vi "Register Worker.vi"(8 "error in (no error)":errorcluster, 10 "Worker":refnum<class "Job Handler.lvclass">, 11 "Mock Worker Processor In":refnum<class "Mock Job Dispatcher.lvclass">) -> (0 "error out":errorcluster, 3 "Mock Worker Processor Out":refnum<class "Mock Job Dispatcher.lvclass">)   [LabVIEW 2020, in "Mock Job Dispatcher.lvclass"]
uses:
  Mock Job Dispatcher.lvclass
  Process Job/Job Handler.lvclass
  Mock Job Dispatcher.lvclass/Mock Job Dispatcher.ctl
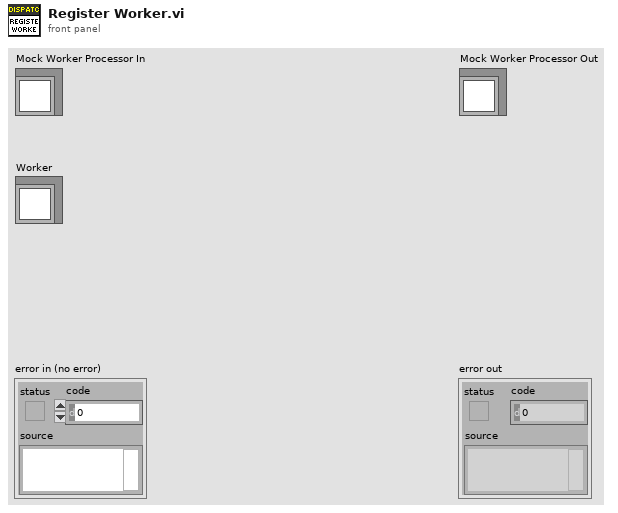
[diagram p1: front panel]
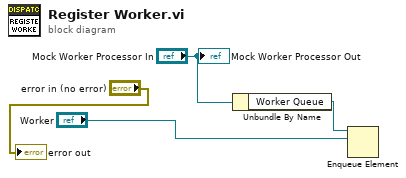
[diagram p0: block diagram]
diagram:
  n1 = Unbundle By Name("Mock Worker Processor In") -> ("Worker Queue"=w3:refnum<queue>)
  n2 = Enqueue Element(queue=w3, element="Worker") -> ()  [unwired: 2 in, 3 out]
  "error out" <- "error in (no error)"
  "Mock Worker Processor Out" <- "Mock Worker Processor In"
